vi "ICtest.vi"() -> ()   [LabVIEW 2015]
uses:
  <vilib>/vision/NI_Vision_Development_Module.lvlib
panel:
  in  "grab":bool
  in  "formats":string(combo)
  in  "devices":string(combo)
  in  "connect":bool
  in  "close":bool
  out "Image":T1(plugin-control)
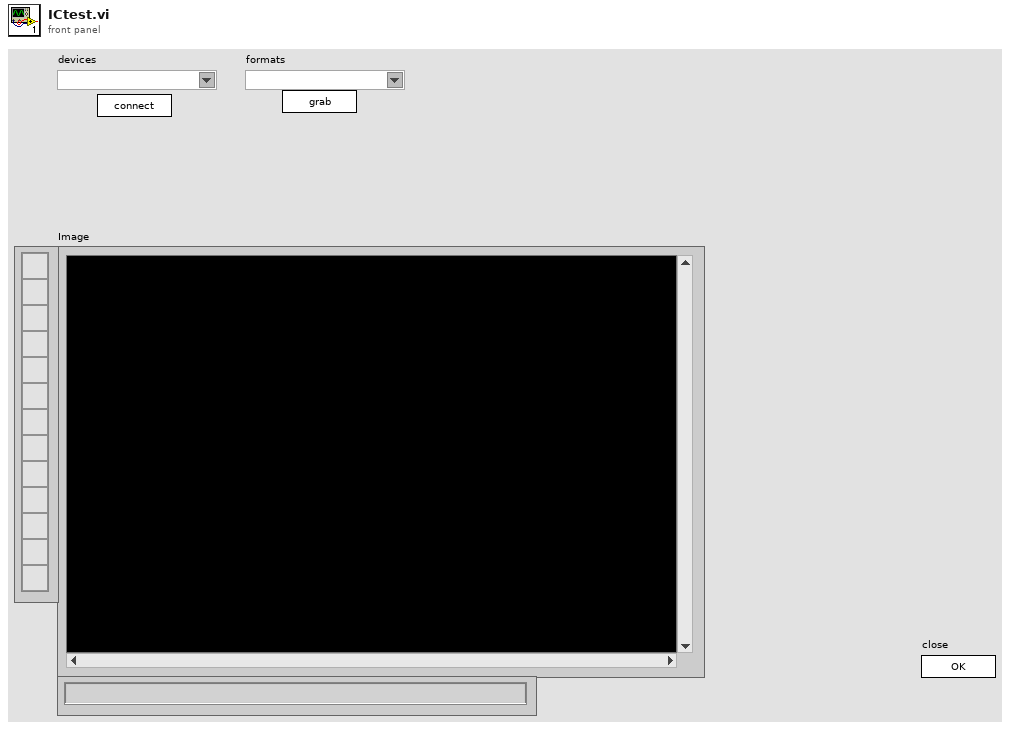
[diagram p1: front panel]
types:
  T1 = typedef "IMAQ Image.ctl" = refnum<image>
  T2 = typedef "Image Type" = u32
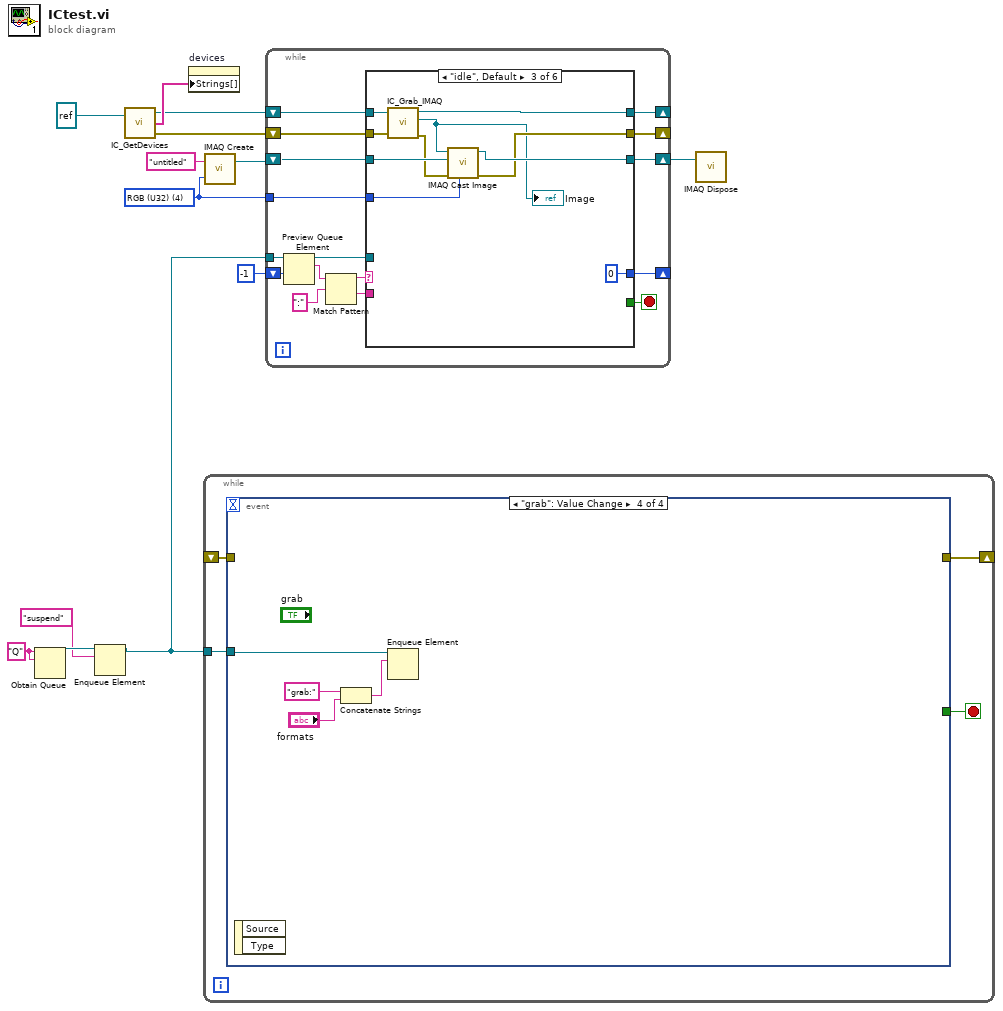
[diagram p0: block diagram]
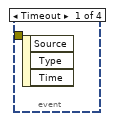
[diagram p2: hidden frame]
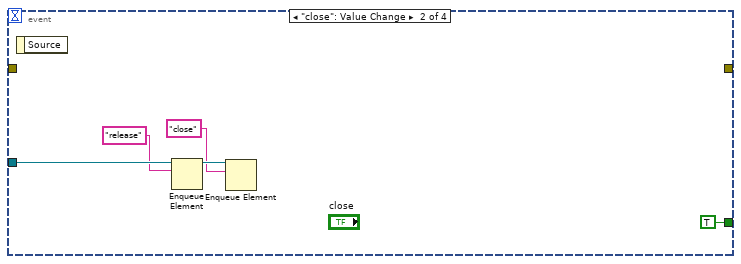
[diagram p3: hidden frame]
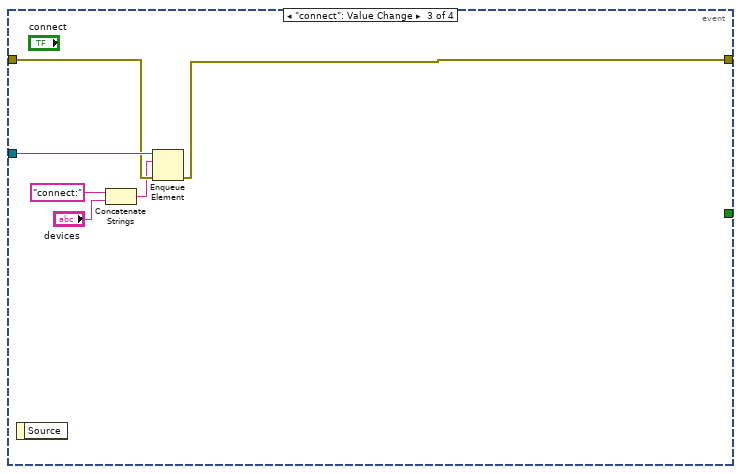
[diagram p4: hidden frame]
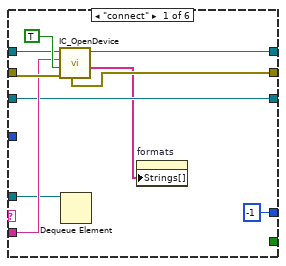
[diagram p5: hidden frame]
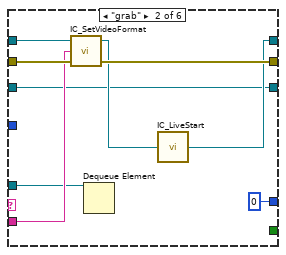
[diagram p6: hidden frame]
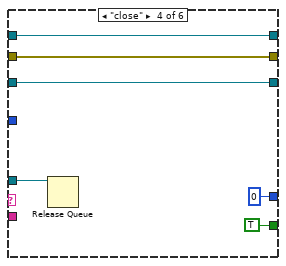
[diagram p7: hidden frame]
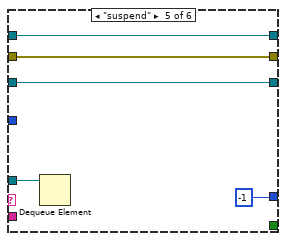
[diagram p8: hidden frame]
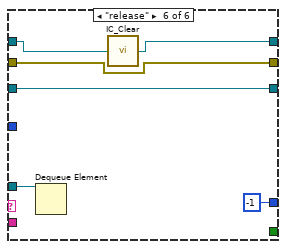
[diagram p9: hidden frame]
diagram:
  w8 = "Q" ("name (unnamed)")
  w11 = T2 4 items=["Grayscale (U8)", "Grayscale (I16)", "Grayscale (SGL)", "Complex (CSG)", "RGB (U32)", "HSL (U32)", "RGB (U64)", "Grayscale (U16)"] ("Image Type")
  n1 = Obtain Queue(name (unnamed)=w8, element data type=w8) -> (queue out=w5:refnum<queue>)  [unwired: 3 in, 2 out]
  n2 = Enqueue Element(queue=w5, element="suspend") -> (queue out=w4:refnum<queue>)  [unwired: 2 in, 2 out]
  n3 = call "IC_GetDevices.vi"("ICImagingControl In"=refnum<k7> refnum ("ICImagingControl")) -> ("ICImagingControl Out"=w7:refnum<k7>, "Devices"=w9:string[], "Error Out"=w6:errorcluster)  [unwired: 1 in]
  n4 = property on="devices" class="CmbBox"("Strings[]"=w9) -> ()  [unwired: 2 in, 2 out]
  n5 = while {
    shift-right: [w15] -> _
    shift-left: _ -> [w16]
    tunnel: w4 -> [w14]
    stop <- w17 stop-if-true
    n6 = event shown="[3] \"grab\": Value Change" {
      selector: _ -> [_ _ _ _]
      dyn-events: _ -> [_ _ _ _]
      timeout: _ -> [_ _ _ _]
      tunnel: [_ TRUE ("close") _ _] -> w17
      tunnel: w16 -> [_ _ w27 _]
      tunnel: [_ _ w26 _] -> w15
      tunnel: w14 -> [_ w22 w28 w29]
      event Timeout {
        n7 = event-data() -> ()  [unwired: 1 in, 3 out]
      }
      event "close": Value Change {
        n8 = event-data() -> ()  [unwired: 1 in, 1 out]
        n9 = Enqueue Element(queue=w22, element="release") -> (queue out=w21:refnum<queue>)  [unwired: 2 in, 2 out]
        n10 = Enqueue Element(queue=w21, element="close") -> ()  [unwired: 2 in, 3 out]
      }
      event "connect": Value Change {
        n11 = event-data() -> ()  [unwired: 1 in, 1 out]
        n12 = Concatenate Strings("connect:" ("string"), "devices") -> (w23:string)
        n13 = Enqueue Element(queue=w28, element=w23, error in (no error)=w27) -> (error out=w26:errorcluster)  [unwired: 1 in, 2 out]
      }
      event "grab": Value Change {
        n14 = event-data() -> ()  [unwired: 1 in, 2 out]
        n15 = Concatenate Strings("grab:" ("string"), "formats") -> (w32:string)
        n16 = Enqueue Element(queue=w29, element=w32) -> ()  [unwired: 2 in, 3 out]
      }
    }
  }
  n17 = call "IMAQ Create"("Image Name"="untitled", "Image Type"=w11) -> ("New Image"=w13:T1)  [unwired: 3 in, 1 out]
  n18 = while {
    shift-right: [w46] -> _
    shift-left: w7 -> [w48]
    shift-right: [w42] -> _
    shift-left: w6 -> [w47]
    tunnel: w11 -> [w44]
    tunnel: w4 -> [w41]
    shift-right: [w43] -> w10
    shift-left: w13 -> [w45]
    shift-right: [w33] -> _
    shift-left: -1 -> [w34]
    stop <- w35 stop-if-true
    n19 = Preview Queue Element(queue=w41, timeout in ms (-1)=w34) -> (queue out=w36:refnum<queue>, element=w40:string)  [unwired: 1 in, 2 out]
    n20 = Match Pattern(string=w40, regular expression=":") -> (before substring=w38:string, after substring=w37:string)  [unwired: 1 in, 2 out]
    n21 = case shown="\"idle\", Default" w38 {
      tunnel: w48 -> [w57 w67 w77 w78 w87 w93]
      tunnel: w47 -> [w56 w66 w76 w80 w86 w91]
      tunnel: [w54 w62 w75 w78 w87 w92] -> w46
      tunnel: w45 -> [w51 w61 w74 w81 w85 w90]
      tunnel: w44 -> [_ _ w73 _ _ _]
      tunnel: [w51 w61 w72 w81 w85 w90] -> w43
      tunnel: [w53 w65 w70 w80 w86 w91] -> w42
      tunnel: w37 -> [w55 w64 _ _ _ _]
      tunnel: w36 -> [w52 w59 _ w82 w84 w94]
      tunnel: [_ _ _ TRUE _ _] -> w35
      tunnel: [-1 0 0 0 -1 -1] -> w33
      frame "connect" {
        n22 = call "IC_OpenDevice.vi"("Error In (no error)"=w56, "Live"=TRUE, "Device"=w55, "ICImagingControl In"=w57) -> ("VideoFormats"=w49:string[], "ICImagingControl Out"=w54:refnum<k7>, "Error Out"=w53:errorcluster)  [unwired: 2 in, 3 out]
        n23 = Dequeue Element(queue=w52) -> ()  [unwired: 2 in, 4 out]
        n24 = property on="formats" class="CmbBox"("Strings[]"=w49) -> ()  [unwired: 2 in, 2 out]
      }
      frame "grab" {
        n25 = call "IC_SetVideoFormat.vi"("Error In (no error)"=w66, "VideoFormat"=w64, "ICImagingControl In"=w67) -> ("Error Out"=w65:errorcluster, "ICImagingControl Out"=w63:refnum<k7>)  [unwired: 1 out]
        n26 = Dequeue Element(queue=w59) -> ()  [unwired: 2 in, 4 out]
        n27 = call "IC_LiveStart.vi"("ICImagingControl 3"=w63) -> ("ICImagingControl 2"=w62:refnum<k7>)
      }
      frame "idle", Default {
        n28 = call "IC_Grab_IMAQ.vi"("ICImagingControl In"=w77, "Error In (no error)"=w76) -> ("ICImagingControl Out"=w75:refnum<k7>, "Image Out"=w68:T1, "Error Out"=w71:errorcluster)  [unwired: 1 in, 1 out]
        "Image" <- w68
        n29 = call "IMAQ Cast Image"("Image Type"=w73, "error in (no error)"=w71, "Image Dst"=w74, "Image Src"=w68) -> ("error out"=w70:errorcluster, "Image Dst Out"=w72:T1)  [unwired: 6 in]
      }
      frame "close" {
        n30 = Release Queue(queue=w82) -> ()  [unwired: 2 in, 3 out]
      }
      frame "suspend" {
        n31 = Dequeue Element(queue=w84) -> ()  [unwired: 2 in, 4 out]
      }
      frame "release" {
        n32 = Dequeue Element(queue=w94) -> ()  [unwired: 2 in, 4 out]
        n33 = call "IC_Clear.vi"("ICImagingControl 2"=w93) -> ("ICImagingControl"=w92:refnum<k7>)
      }
    }
  }
  n34 = call "IMAQ Dispose"("Image"=w10) -> ()  [unwired: 5 in, 1 out]
